vi "Dashboard Main.vi"() -> ()   [LabVIEW 2014]
uses:
  <vilib>/event_ctls.llb/eventvkey.ctl
  <vilib>/Rock Robotics/WPI/Dashboard/WPI_DashboardLogging Global.vi
  <vilib>/Rock Robotics/Network Tables/SD Write String.vi
  <vilib>/Rock Robotics/Network Tables/SD Read Number.vi
  <vilib>/Rock Robotics/Network Tables/SD Read Boolean.vi
  <vilib>/Rock Robotics/Network Tables/SD Write Boolean.vi
  <vilib>/Utility/config.llb/Write Key (String).vi
  <vilib>/Utility/config.llb/Write Key (I32).vi
  <vilib>/Utility/config.llb/NI_LVConfig.lvlib
panel:
  in  "TCP":refnum<k5>
  in  "Rec Mode":enum32{"Stop", "Record", "Playback"}(radio)
  in  "Vision":u16(ring) items=["Camera Off", "USB Camera SW", "USB Camera HW", "IP Camera"]
  out "Camera IP":string
  out "Image Message":string="Timeout in Camera Communications"
  in  "Dashboard Tab":T1(tab)
  in  "PID":bool
  in  "Camera Settings":T2={"Frame Rate"=30, "Compression"=30, "Size"=1} {"Frame Rate" scale=1.0..30.0; "Size" items=["640x480", "320x240", "160x120"]}
  out "MotorChart R":cluster{"Numeric":dbl, "Numeric":dbl}(graph)
  out "MotorChart L":T3(graph)
  out "MotorSliders R":cluster{"MotorSlide1":dbl, "MotorSlide2":dbl} {"MotorSlide2" scale=-1.0..1.0 scale format="%#_2e"; "MotorSlide1" scale=-1.0..1.0 scale format="%#_2e"}
  out "MotorSliders L":T4 {"MotorSlide4 2" scale=0.0..14.0 scale format="%#_2e"; "MotorSlide2" scale=-1.0..1.0 scale format="%#_2e"; "MotorSlide1" scale=-1.0..1.0 scale format="%#_2e"}
  out "Gyro":dbl(knob) scale=0.0..360.0
  out "JS1 Z":dbl(slide) scale=-1.0..1.0 scale format="%#_2e"
  out "JS1 Graph":cluster{"X":dbl, "Y":dbl}[](graph)
  out "JS1 Buttons":T5
  out "JS2 Z":dbl(slide) scale=-1.0..1.0 scale format="%#_2e"
  out "JS2 Graph":cluster{"X":dbl, "Y":dbl}[](graph)
  out "JS2 Buttons":T5
  out "Mode":T6(ring)=enum."Auto Disabled"
  in  "DB Camera Config":bool
  out "fps":dbl format="%#.1g"
  out "Mbps":dbl format="%#.1g"
  out "Mbps 2":bool
  out "Manual Forks?":bool
  out "PID?":bool
  in  "DB/String 9":string
  in  "DB/String 8":string
  in  "DB/String 7":string
  in  "DB/String 6":string
  in  "DB/String 5":string
  in  "DB/String 4":string
  in  "DB/String 3":string
  in  "DB/String 2":string
  in  "DB/String 1":string
  in  "DB/String 0":string
  in  "DB/Slider 0":dbl(slide) scale=0.0..5.0
  in  "DB/Slider 1":dbl(slide) scale=0.0..5.0
  in  "DB/Slider 2":dbl(slide) scale=0.0..5.0
  in  "DB/Slider 3":dbl(slide) scale=0.0..5.0
  out "DB/LED 3":bool
  out "DB/LED 2":bool
  out "DB/LED 1":bool
  out "DB/LED 0":bool
  in  "DB/Button 3":bool
  in  "DB/Button 2":bool
  in  "DB/Button 1":bool
  in  "DB/Button 0":bool caption="New Name"
  in  "AUTO Modes":T7(tab)
  in  "AUTO?":bool=TRUE
  in  "MODE":bool
  out "Totes":bool
  in  "Ring":u16(ring) items=["Left/Tote", "Left/Bin"]
  in  "Ring 2":u16(ring) items=["Center/Tote", "Center/Bin"]
  in  "Ring 3":u16(ring) items=["Right/Tote", "Right/Bin", "Right/HPS"]
  out "AUTO Zone":bool
  in  "Mode":u16(ring) items=["Drive into AUTO Zone", "Nothing"]
  in  "Test Slider":dbl(slide) scale=0.0..100.0 scale format="%#_3g"
  in  "On/Off":bool caption="Solenoid"
  in  "Test Name":u16(ring) items=["Select the test to run...", "Example Test", "-------------------------------", "List of tests is built in robot code.", "Replace with your own automated tests."]
  in  "Test Tree":string(tree)
  in  "Motor":cluster{"Value":dbl, "Enable":bool} {"Value" scale=-1.0..1.0 scale format="%#_3g"}
  out "Progress":T8 {"Test Progress" scale=0.0..100.0}
  in  "Rev/Fwd":cluster{"Forward":bool, "Reverse":bool}
  in  "Test Ring":u16(ring) items=["Monochrome", "Color"]
  in  "Listbox":i32(listbox)
  out "Tree":string(tree)
  out "Camera Image":T9(plugin-control)
  out "Boolean":bool
  # "Left"
  # "Front"
  # "Right"
  # "Battery"
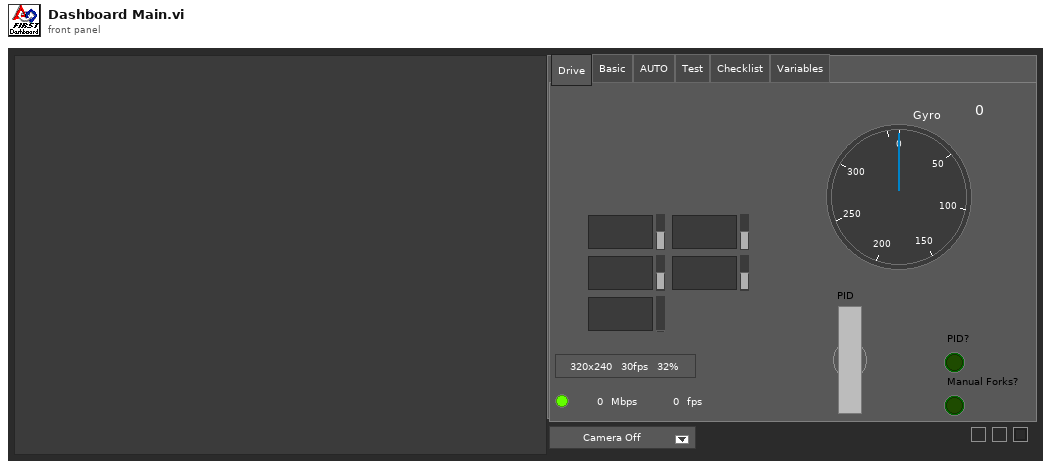
[diagram p1: front panel]
types:
  T1 = enum32{"Drive", "Basic", "AUTO", "Test", "Checklist", "Variables"}
  T2 = cluster{"Frame Rate":i32, "Compression":i32, "Size":u16}
  T3 = cluster{"Numeric":dbl, "Numeric":dbl, "Battery V":dbl}
  T4 = cluster{"MotorSlide1":dbl, "MotorSlide2":dbl, "MotorSlide4 2":dbl}
  T5 = cluster{bool, bool, bool, bool, bool, bool, bool, bool, bool, bool, bool, bool}
  T6 = enum8{"Tele-Op Disabled", "Tele-Op Enabled", "Auto Disabled", "Auto Enabled", "Test Disabled", "Test Enabled", "Disconnected", "No Code", "E-Stop"}
  T7 = enum32{"NEW USE THIS MODE", "Left", "Center", "Right", "Open Area", "Landfill"}
  T8 = cluster{"Test Progress":u8, "Test Progress Text":string}
  T9 = typedef "IMAQ Image.ctl" = refnum<image>
  T10 = enum32{"Drive", "Basic", "Custom", "Test", "Checklist", "Variables"}
  T11 = typedef "Image Type" = u32
  T12 = cluster{"Camera Image":refnum<vi>, "Dashboard Tab":refnum<vi>, "Boolean":refnum<vi>, "Vision":refnum<vi>, "Rec Mode":refnum<vi>, "Test Slider":refnum<vi>, "On/Off ":refnum<vi>, "Test Ring":refnum<vi>, "Rev/Fwd":refnum<vi>, "Test Name":refnum<vi>, "Motor":refnum<vi>, "Progress":refnum<vi>, "CheckList":refnum<vi>, "Tree":refnum<vi>, "Test Tree":refnum<vi>}
  T13 = cluster{"Error Strings":string, "Disable Counts":cluster{u16, u16}, "Rail Faults":cluster{u16, u16, u16}, "Robot IP":string, "DB Mode":u8, "Event Info":cluster{"Name":string, "Type":u8, "Number":u16, "Replay":u8}, "Camera Addr":string}
  T14 = cluster{"Storage":cluster{"Disk Free":u64, "RAM Block":u32, "RAM free":u32}, "CPU Utilization":cluster{"CPU % ISR":sgl, "CPU % Time Crit":sgl, "CPU % Timed Str":sgl, "CPU % High":sgl, "CPU % Above":sgl, "CPU % Normal":sgl, "CPU % Low":sgl}, "CAN":cluster{"% Bus Utilization":sgl, "Bus Off Cnt":u32, "TX_FIFO Full Cnt":u32, "Receive Error Cnt":u8, "Transmit Error Cnt":u8}, "HID":cluster{"HID Outputs":u32, "Rumble Low":u16, "Rumble High":u16}[]}
  T15 = cluster{"Status bits":cluster{"Test Mode":bool, "Autonomous":bool, "Enabled":bool, "Code Start":bool, "Brownout":bool, "Reserved 2":bool, "Reserved 3":bool, "E-Stop":bool}, "Code Trace":cluster{"Disabled":bool, "TeleOp":bool, "Auto":bool, "Test":bool}, "Controller Type":enum16{"unknown", "cRIO", "roboRio"}, "Code?":enum16{"unknown", "noCode", "code"}, "Battery V":dbl}
  T16 = cluster{"Control Bits":cluster{"TestMode":bool, "Autonomous":bool, "Enabled":bool, "FMS Present":bool, bool, bool, bool, "E-Stop":bool}, "Team Station ":u8, "Countdown":sgl, "Joystick Values":cluster{"Axes":dbl[], "Buttons":bool[], "POVs":i16[]}[]}
  T17 = cluster{"Axes":dbl[], "Buttons":bool[], "POVs":i16[]}[]
  T18 = cluster{"Axes":dbl[], "Buttons":bool[], "POVs":i16[]}
  T19 = cluster{"Buttons[0]":bool, "Buttons[1]":bool, "Buttons[2]":bool, "Buttons[3]":bool, "Buttons[4]":bool, "Buttons[5]":bool, "Buttons[6]":bool, "Buttons[7]":bool, "Buttons[8]":bool, "Buttons[9]":bool, "Buttons[10]":bool, "Buttons[11]":bool}
  T20 = typedef "NI_LVConfig.lvlib/Config Data RefNum.ctl" = refnum<k1>
  T21 = cluster{"Operation":enum16{"Update", "Clear"}, "Color Box":u32}[]
  T22 = typedef "eventvkey.ctl" = enum16{"ASCII", "Enter", "Return", "Shift", "Ctrl", "Alt", "Cmd", "Opt", "Caps", "NumLock", "Clear", "Break", "Up", "Down", "Left", "Right", "Insert", "Delete", "Home", "End", "PageUp", "PageDown", "Escape", "Help", "Pause", "ScrollLock", "F1", "F2", "F3", "F4", "F5", "F6", "F7", "F8", "F9", "F10", "F11", "F12", "F13", "F14", "F15", "F16", "F17", "F18", "F19", "F20", "F21", "F22", "F23", "F24", "Play", "VolumeUp", "VolumeDown", "Mute", "Two Byte Char"}
  T23 = cluster{"Image Size":bool, "Image Type":bool, "Pixel Value":bool, "ROI Information":bool, "Zoom Factor":bool}
  T24 = enum8{"Enabled", "Disabled", "Disabled and Grayed Out"}
  T25 = cluster{"Operation":enum16{"Update", "Clear"}, "Color Box":u32}
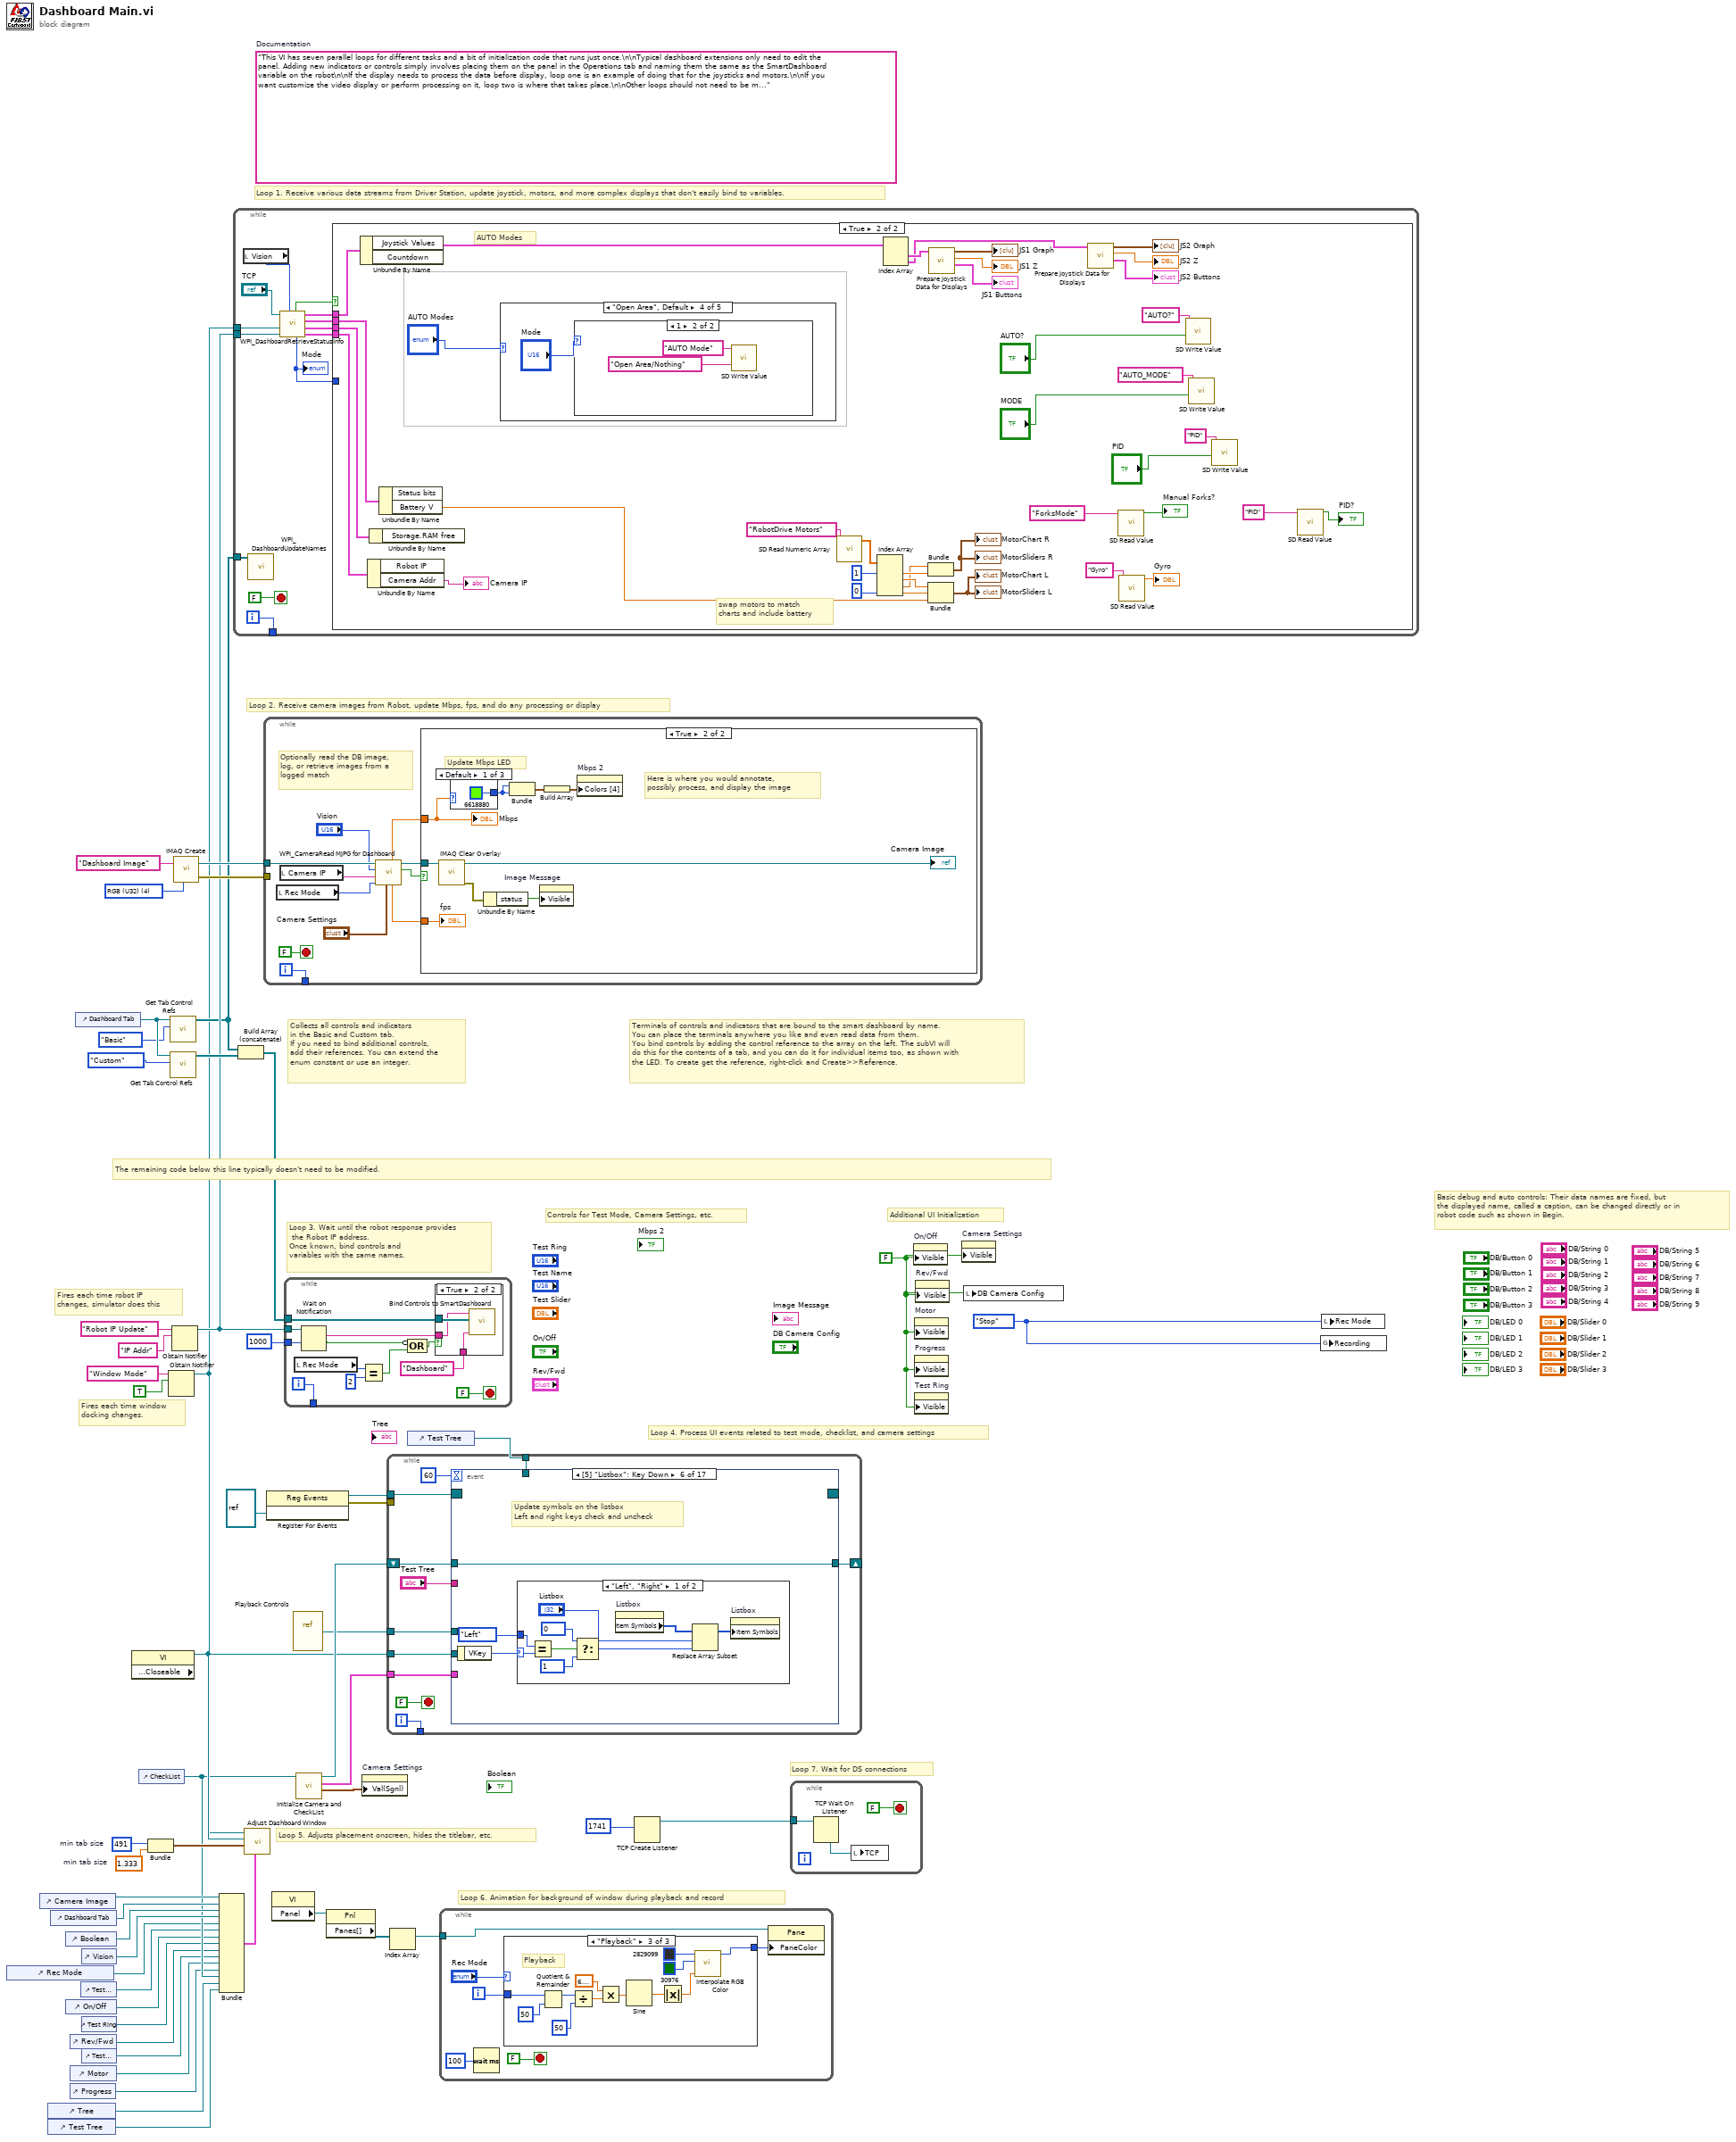
[diagram p0: block diagram]
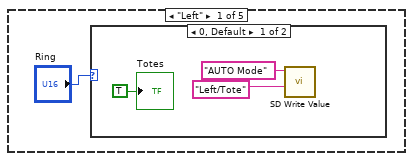
[diagram p3: hidden frame]
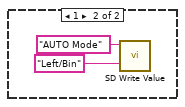
[diagram p4: hidden frame]
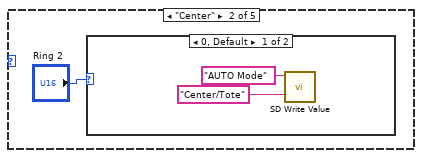
[diagram p5: hidden frame]
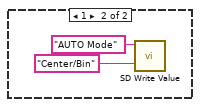
[diagram p6: hidden frame]
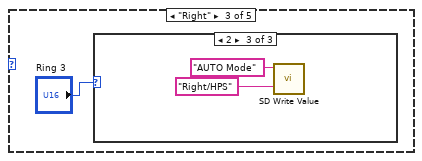
[diagram p7: hidden frame]
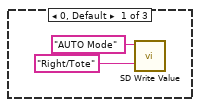
[diagram p8: hidden frame]
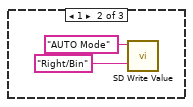
[diagram p9: hidden frame]
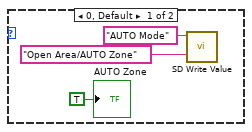
[diagram p10: hidden frame]
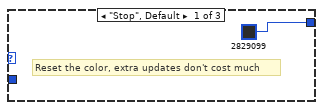
[diagram p12: hidden frame]
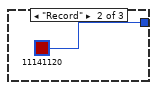
[diagram p13: hidden frame]
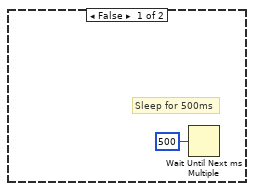
[diagram p15: hidden frame]
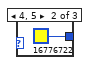
[diagram p16: hidden frame]
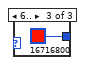
[diagram p17: hidden frame]
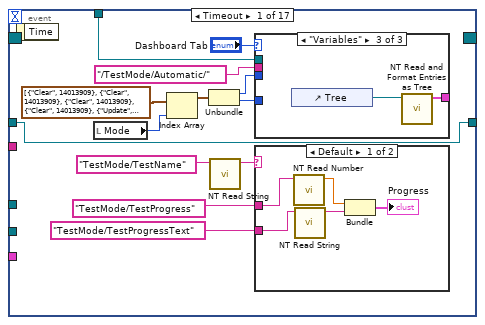
[diagram p18: hidden frame]
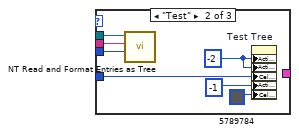
[diagram p20: hidden frame]
diagram:
  w24 = 491  # min tab size
  w23 = 1.333  # min tab size
  w32 = enum32{"Stop", "Record", "Playback"}."Stop" ("Rec Mode")
  w6 = FALSE ("Visible")
  (unwired) "This VI has seven parallel loops for different tasks and a bit of initialization code that runs just once.\n\nTypical dashboard extensions only need to edit the panel. Adding new indicators or controls simply involves placing them on the panel in the Operations tab and naming them the same as the SmartDashboard variable on the robot\n\nIf the display needs to process the data before display, loop one is an example of doing that for the joysticks and motors.\n\nIf you want customize the video display or perform processing on it, loop two is where that takes place.\n\nOther loops should not need to be modified. They are pretty standard, and document the task they perform."  # Documentation
  w52 = T11 4 items=["Grayscale (U8)", "Grayscale (I16)", "Grayscale (SGL)", "Complex (CSG)", "RGB (U32)", "HSL (U32)", "RGB (U64)"] ("Image Type")
  # "Loop 7. Wait for DS connections"
  # "Basic debug and auto controls: Their data names are fixed, but\nthe displayed name, called a caption, can be changed directly or in\nrobot code such as shown in Begin."
  # "Controls for Test Mode, Camera Settings, etc."
  # "Additional UI Initialization"
  # "Loop 6. Animation for background of window during playback and record"
  # "Fires each time robot IP\nchanges, simulator does this"
  # "Fires each time window\ndocking changes."
  # "Collects all controls and indicators\nin the Basic and Custom tab.\nIf you need to bind additional controls,\nadd their references. You can extend the\nenum constant or use an integer."
  # "The remaining code below this line typically doesn't need to be modified."
  # "Loop 4. Process UI events related to test mode, checklist, and camera settings"
  # "Terminals of controls and indicators that are bound to the smart dashboard by name.\nYou can place the terminals anywhere you like and even read data from them.\nYou bind controls by adding the control reference to the array on the left. The subVI will\ndo this for the contents of a tab, and you can do it for individual items too, as shown with\nthe LED. To create get the reference, right-click and Create>>Reference."
  # "Loop 3. Wait until the robot response provides\n the Robot IP address.\nOnce known, bind controls and\nvariables with the same names."
  # "Loop 5. Adjusts placement onscreen, hides the titlebar, etc."
  # "Loop 1. Receive various data streams from Driver Station, update joystick, motors, and more complex displays that don't easily bind to variables."
  # "Loop 2. Receive camera images from Robot, update Mbps, fps, and do any processing or display"
  n1 = control-ref of="Rec Mode"() -> (w12:refnum<vi>)
  n2 = control-ref of="Camera Image"() -> (w27:refnum<vi>)
  n3 = control-ref of="Tree"() -> (w16:refnum<vi>)
  n4 = control-ref of="Test Tree"() -> (w15:refnum<vi>)
  n5 = control-ref of="Dashboard Tab"() -> (w26:refnum<vi>)
  n6 = control-ref of="Boolean"() -> (w21:refnum<vi>)
  n7 = control-ref of="On/Off"() -> (w10:refnum<vi>)
  n8 = control-ref of="Progress"() -> (w7:refnum<vi>)
  n9 = control-ref of="Rev/Fwd"() -> (w8:refnum<vi>)
  n10 = control-ref of="Motor"() -> (w13:refnum<vi>)
  n11 = control-ref of="Dashboard Tab"() -> (w30:refnum<vi>)
  n12 = control-ref of="Test Slider"() -> (w11:refnum<vi>)
  n13 = control-ref of="Vision"() -> (w25:refnum<vi>)
  n14 = control-ref of="Test Ring"() -> (w9:refnum<vi>)
  n15 = control-ref of="Test Name"() -> (w14:refnum<vi>)
  n16 = property class="VI" props=["Front Panel.Closeable"]() -> (reference out=w31:refnum<vi>)  [unwired: 2 in, 2 out]
  n17 = control-ref of="CheckList"() -> (w17:refnum<vi>)
  n18 = Bundle("min tab size"=w24, "min tab size"=w23) -> (w22:cluster{"min tab size":i32, "min tab size":dbl})  [unwired: 1 in]
  n19 = Obtain Notifier(name (unnamed)="Window Mode", notification data type=TRUE) -> (notifier out=w3:refnum<notifier>)  [unwired: 2 in, 2 out]
  n20 = call <vilib>:"Get Tab Control Refs.vi"("Page Index"=T10."Basic" ("Dashboard Tab"), "TabControl in"=w30) -> ("ControlsOnPage"=w4:refnum<vi>[])  [unwired: 9 in]
  n21 = call <vilib>:"Get Tab Control Refs.vi"("Page Index"=T10."Custom" ("Dashboard Tab"), "TabControl in"=w30) -> ("ControlsOnPage"=w29:refnum<vi>[])  [unwired: 9 in]
  n22 = Obtain Notifier(name (unnamed)="Robot IP Update", notification data type="IP Addr" ("name (unnamed)")) -> (notifier out=w5:refnum<notifier>)  [unwired: 2 in, 2 out]
  n23 = call "IMAQ Create"("Image Name"="Dashboard Image", "Image Type"=w52) -> ("New Image"=w50:T9, "error out"=w49:errorcluster)  [unwired: 2 in, 1 out]
  n24 = Bundle("Camera Image"=w27, "Dashboard Tab"=w26, "Boolean"=w21, "Vision"=w25, "Rec Mode"=w12, "Test Slider"=w11, "On/Off"=w10, "Test Ring"=w9, "Rev/Fwd"=w8, "Test Name"=w14, "Motor"=w13, "Progress"=w7, "CheckList"=w17, "Tree"=w16, "Test Tree"=w15) -> (w18:T12)  [unwired: 1 in]
  n25 = while {
    tunnel: [w64] -> _
    tunnel: w5 -> [w58]
    tunnel: w4 -> [w57]
    tunnel: w3 -> [w53]
    i -> [w64]
    stop <- FALSE stop-if-true
    n26 = local read "Vision"() -> (w55:u16)
    n27 = call <vilib>:"WPI_DashboardUpdateNames.vi"("Controls on Tab"=w57) -> ()  [unwired: 11 in]
    n28 = call <vilib>:"WPI_DashboardRetrieveStatusInfo.vi"("Vision"=w55, "Binding Refnum"=w58, "Window Mode Notifier"=w53, "TCP Cnx"="TCP") -> ("Power and Errors"=w59:T13, "Robot Metrics"=w62:T14, "Status Info"=w63:T15, "Control Info"=w60:T16, "Robot Mode"=w56:T6, "Process?"=w61:bool)  [unwired: 2 in]
    "Mode" <- w56
    n29 = case shown="True" w61 {
      tunnel: w63 -> [_ w103]
      tunnel: w62 -> [_ w102]
      tunnel: w60 -> [_ w101]
      tunnel: w59 -> [_ w100]
      tunnel: w56 -> [_ _]
      frame False {
      }
      frame True {
        # "AUTO Modes"
        # "swap motors to match\ncharts and include battery"
        n30 = Unbundle By Name(w101) -> ("Joystick Values"=w88:T17)  [unwired: 1 out]
        n31 = Unbundle By Name(w100) -> ("Camera Addr"=→"Camera IP":string)  [unwired: 1 out]
        n32 = Unbundle By Name(w102) -> ()  [unwired: 1 out]
        n33 = Unbundle By Name(w103) -> ("Battery V"=w89:dbl)  [unwired: 1 out]
        n34 = case shown="\"Open Area\", Default" "AUTO Modes" {
          frame "Left" {
            n35 = case shown="0, Default" "Ring" {
              frame 0, Default {
                n36 = call-poly <vilib>:"SD Write Value.vi"("String"="Left/Tote", "Name"="AUTO Mode") -> ()  [unwired: 8 in, 2 out]
                "Totes" <- TRUE ("Totes")
              }
              frame 1 {
                n37 = call-poly <vilib>:"SD Write Value.vi"("String"="Left/Bin", "Name"="AUTO Mode") -> ()  [unwired: 8 in, 2 out]
              }
            }
          }
          frame "Center" {
            n38 = case shown="0, Default" "Ring 2" {
              frame 0, Default {
                n39 = call-poly <vilib>:"SD Write Value.vi"("String"="Center/Tote", "Name"="AUTO Mode") -> ()  [unwired: 8 in, 2 out]
              }
              frame 1 {
                n40 = call-poly <vilib>:"SD Write Value.vi"("String"="Center/Bin", "Name"="AUTO Mode") -> ()  [unwired: 8 in, 2 out]
              }
            }
          }
          frame "Right" {
            n41 = case shown="2" "Ring 3" {
              frame 0, Default {
                n42 = call-poly <vilib>:"SD Write Value.vi"("String"="Right/Tote", "Name"="AUTO Mode") -> ()  [unwired: 8 in, 2 out]
              }
              frame 1 {
                n43 = call-poly <vilib>:"SD Write Value.vi"("String"="Right/Bin", "Name"="AUTO Mode") -> ()  [unwired: 8 in, 2 out]
              }
              frame 2 {
                n44 = call-poly <vilib>:"SD Write Value.vi"("String"="Right/HPS", "Name"="AUTO Mode") -> ()  [unwired: 8 in, 2 out]
              }
            }
          }
          frame "Open Area", Default {
            n45 = case shown="1" "Mode" {
              frame 0, Default {
                n46 = call-poly <vilib>:"SD Write Value.vi"("String"="Open Area/AUTO Zone", "Name"="AUTO Mode") -> ()  [unwired: 8 in, 2 out]
                "AUTO Zone" <- TRUE ("AUTO Zone")
              }
              frame 1 {
                n47 = call-poly <vilib>:"SD Write Value.vi"("String"="Open Area/Nothing", "Name"="AUTO Mode") -> ()  [unwired: 8 in, 2 out]
              }
            }
          }
          frame "Landfill" {
          }
        }
        n48 = call <vilib>:"SD Read Numeric Array.vi"("Name"="RobotDrive Motors") -> ("Numeric Array"=w91:dbl[])  [unwired: 8 in, 2 out]
        n49 = Index Array(array=w91, index #1=1, index #4=0) -> (element #1=w95:dbl, element #2=w96:dbl, element #3=w94:dbl, element #4=w99:dbl)  [unwired: 2 in]
        n50 = Index Array(array=w88) -> (element #1=w87:T18, element #2=w82:T18)  [unwired: 2 in]
        n51 = Bundle("Numeric"=w94, "Numeric"=w95) -> (→"MotorChart R" →"MotorSliders R":cluster{"Numeric":dbl, "Numeric":dbl})  [unwired: 1 in]
        n52 = Bundle("Numeric"=w96, "Numeric"=w99, "Battery V"=w89) -> (→"MotorChart L" →"MotorSliders L":T3)  [unwired: 1 in]
        n53 = call "Prepare Joystick Data for Displays.vi"("Joystick Values"=w87) -> ("Buttons"=→"JS1 Buttons":T19, "Z Axis"=→"JS1 Z":dbl, "Cartesian Data"=→"JS1 Graph":cluster{"X axis":dbl, "X axis":dbl}[])  [unwired: 8 in]
        n54 = call "Prepare Joystick Data for Displays.vi"("Joystick Values"=w82) -> ("Buttons"=→"JS2 Buttons":T19, "Z Axis"=→"JS2 Z":dbl, "Cartesian Data"=→"JS2 Graph":cluster{"X axis":dbl, "X axis":dbl}[])  [unwired: 8 in]
        n55 = call-poly <vilib>:"SD Read Value.vi"("Name"="ForksMode") -> ("Boolean"=→"Manual Forks?":bool)  [unwired: 8 in, 2 out]
        n56 = call-poly <vilib>:"SD Read Value.vi"("Name"="Gyro") -> ("Numeric"=→"Gyro":dbl)  [unwired: 8 in, 2 out]
        n57 = call-poly <vilib>:"SD Write Value.vi"("Boolean"="AUTO?", "Name"="AUTO?") -> ()  [unwired: 8 in, 2 out]
        n58 = call-poly <vilib>:"SD Write Value.vi"("Boolean"="MODE", "Name"="AUTO_MODE") -> ()  [unwired: 8 in, 2 out]
        n59 = call-poly <vilib>:"SD Write Value.vi"("Boolean"="PID", "Name"="PID") -> ()  [unwired: 8 in, 2 out]
        n60 = call-poly <vilib>:"SD Read Value.vi"("Name"="PID") -> ("Boolean"=→"PID?":bool)  [unwired: 8 in, 2 out]
      }
    }
  }
  n61 = Build Array (concatenate)(w4, w29) -> (w28:refnum<vi>[])
  n62 = call "Adjust Dashboard Window.vi"("Sizing Refnums"=w18, "Size Constraints"=w22, "VI"=w31, "Notifier in"=w3) -> ()  [unwired: 8 in]
  n63 = while {
    tunnel: w50 -> [w136]
    tunnel: w49 -> [_]
    tunnel: [w137] -> _
    i -> [w137]
    stop <- FALSE stop-if-true
    # "Optionally read the DB image,\nlog, or retrieve images from a\nlogged match"
    n64 = local read "Rec Mode"() -> (w130:enum32{"Stop", "Record", "Playback"})
    n65 = local read "Camera IP"() -> (w128:string)
    n66 = call <vilib>:"WPI_CameraRead MJPG for Dashboard.vi"("Camera Settings"="Camera Settings", "Rec Mode"=w130, "Camera IP"=w128, "Camera Mode"="Vision", "Refnum in"=w136) -> ("Active"=w134:bool, "Refnum out"=w135:T9, "FPS"=w133:dbl, "Bandwidth (Mbps)"=w132:dbl)  [unwired: 3 in]
    n67 = case shown="True" w134 {
      tunnel: w135 -> [_ w143]
      tunnel: w132 -> [_ w142]
      tunnel: w133 -> [_ w140]
      frame False {
        # "Sleep for 500ms"
        n68 = Wait Until Next ms Multiple(millisecond multiple=u32 500) -> ()  [unwired: 1 out]
      }
      frame True {
        # "Here is where you would annotate,\npossibly process, and display the image"
        # "Update Mbps LED"
        n69 = call "IMAQ Clear Overlay"("Image"=w143) -> ("error out"=w147:errorcluster, "Image Out"=→"Camera Image":T9)  [unwired: 2 in, 7 out]
        n70 = case shown="Default" w142 {
          tunnel: [u32 6618880 ("Color Box") u32 16776722 ("Color Box") u32 16716800 ("Color Box")] -> w144
          frame Default {
          }
          frame 4, 5 {
          }
          frame 6.. {
          }
        }
        n71 = Unbundle By Name(w147) -> ("status"=w148:bool)
        n72 = Bundle("Color Box"=w144, "Color Box"=w144) -> (w146:cluster{"Color Box":u32, "Color Box":u32})  [unwired: 1 out]
        n73 = property on="Image Message" class="Str"("Visible"=w148) -> ()  [unwired: 2 in, 2 out]
        n74 = Build Array(w146) -> (w145:cluster{"Color Box":u32, "Color Box":u32}[])
        n75 = property on="Mbps 2" class="Bool (strict)"("Colors [4]"=w145) -> ()  [unwired: 2 in, 2 out]
        "Mbps" <- w142
        "fps" <- w140
      }
    }
  }
  n76 = register-events(refnum<vi> refnum) -> (reference out=w36:refnum<event-registration>, error out=w35:errorcluster)  [unwired: 2 in]
  n77 = property class="VI"() -> ("Panel"=w39:refnum<vi>)  [unwired: 2 in, 2 out]
  n78 = while {
    tunnel: w28 -> [w163]
    tunnel: w5 -> [w161]
    tunnel: [w159] -> _
    tunnel: u32 1000 ("milliseconds to wait") -> [w158]
    i -> [w159]
    stop <- FALSE stop-if-true
    n79 = local read "Rec Mode"() -> (w154:enum32{"Stop", "Record", "Playback"})
    n80 = Wait on Notification(notifier=w161, timeout in ms (-1)=w158) -> (notification=w160:string, timed out?=w156:bool)  [unwired: 2 in, 2 out]
    n81 = Equal?(x=w154, y=u16 2 ("Rec Mode")) -> (x = y?=w155:bool)
    n82 = Compound Arithmetic op=OR(invert w156, w155) -> (w157:bool)
    n83 = case shown="True" w157 {
      tunnel: w163 -> [_ w166]
      tunnel: w160 -> [_ w165]
      tunnel: "Dashboard" -> [_ w164]
      frame False {
      }
      frame True {
        n84 = call <vilib>:"Bind Controls to SmartDashboard.vi"("Client Name"=w164, "Bound Control Refs"=w166, "Server IP Address"=w165) -> ()  [unwired: 9 in]
      }
    }
  }
  n85 = vi-ref "Playback Controls.vi"() -> (w37:refnum<vi>)
  n86 = call "Initialize Camera and CheckList.vi"("ListBox in"=w17) -> ("Cluster"=w43:cluster{"value":i32, "value":i32, "index":i32}, "Array"=w44:cluster{string[]}[], "File Refnum"=w42:T20)  [unwired: 8 in]
  n87 = property class="Pnl"(reference=w39) -> ("Panes[]"=w40:refnum<vi>[])  [unwired: 1 in, 2 out]
  n88 = property on="Camera Settings" class="Clust (strict)"("Val(Sgnl)"=w43) -> ()  [unwired: 2 in, 2 out]
  n89 = Index Array(array=w40) -> (element=w38:refnum<vi>)  [unwired: 1 in]
  n90 = control-ref of="Test Tree"() -> (w41:refnum<vi>)
  n91 = while {
    tunnel: w44 -> [w174]
    shift-right: [w173] -> _
    shift-left: w42 -> [w172]
    tunnel: [w171] -> _
    tunnel: w41 -> [w170]
    tunnel: w37 -> [w169]
    tunnel: w36 -> [w168]
    tunnel: w35 -> [_]
    tunnel: w31 -> [w167]
    i -> [w171]
    stop <- FALSE stop-if-true
    n92 = event shown="[5] \"Listbox\": Key Down" {
      selector: w168 -> [_ _ _ _ _ _ _ _ _ _ _ _ _ _ _ _ _]
      dyn-events: [_ _ _ _ _ _ _ _ _ _ _ _ _ w412 _ _ _] -> _
      timeout: u32 60 ("milliseconds to wait") -> [_ _ _ _ _ _ _ _ _ _ _ _ _ _ _ _ _]
      tunnel: w170 -> [w186 _ _ _ _ _ _ _ _ _ _ _ _ _ _ _ _]
      tunnel: "Test Tree" -> [_ _ _ _ _ _ _ _ w381 w389 w391 w395 w403 _ _ _ _]
      tunnel: w174 -> [_ w208 _ _ _ _ w345 w375 _ _ _ _ _ _ _ _ _]
      tunnel: [w182 w207 w306 w311 w319 w331 w344 w368 w380 w387 w390 w394 w402 w414 w428 w429 w439] -> w173
      tunnel: w172 -> [w182 w207 w306 w311 w319 w331 w343 w368 w380 w387 w390 w394 w402 w414 w428 w429 w439]
      tunnel: w169 -> [_ _ _ _ _ _ _ _ _ _ _ _ _ w415 _ w432 _]
      tunnel: w167 -> [_ _ _ _ _ _ _ _ _ _ _ _ _ w410 _ _ _]
      event Timeout {
        n93 = event-data() -> ()  [unwired: 1 in, 1 out]
        n94 = local read "Mode"() -> (w185:T6)
        n95 = Index Array(array=T21 [{"Operation"=enum."Clear", "Color Box"=14013909}, {"Operation"=enum."Clear", "Color Box"=14013909}, {"Operation"=enum."Clear", "Color Box"=14013909}, {"Operation"=enum."Clear", "Color Box"=14013909}, {"Operation"=enum."Update", "Color Box"=14013909}, {"Operation"=enum."Update", "Color Box"=16777215}, {"Operation"=enum."Clear", "Color Box"=14013909}, {"Operation"=enum."Clear", "Color Box"=14013909}, {"Operation"=enum."Clear", "Color Box"=14013909}], index=w185) -> (element=w180:T25)
        n96 = Unbundle(w180) -> ("Operation"=w179:enum16{"Update", "Clear"}, "Color Box"=w178:u32)
        n97 = call <vilib>:"NT Read String.vi"("Name"="TestMode/TestName") -> ("String"=w189:string)  [unwired: 9 in, 1 out]
        n98 = case shown="\"Variables\"" "Dashboard Tab" {
          tunnel: w186 -> [_ w197 _]
          tunnel: "/TestMode/Automatic/" ("Name Pattern") -> [_ w196 _]
          tunnel: w179 -> [_ w195 _]
          tunnel: [_ _ w199] -> _
          tunnel: w178 -> [_ w191 _]
          frame "AUTO", Default {
          }
          frame "Test" {
            w194 = -2 ("Active Item:Row Number")
            n99 = call <vilib>:"NT Read and Format Entries as Tree.vi"("Operation"=w195, "Name Pattern"=w196, "Tree Refnum"=w197) -> ()  [unwired: 7 in, 2 out]
            n100 = property on="Test Tree" class="Tree (strict)"("Active Item Row Number"=w194, "ActiveColNum"=w194, "CellBG"=w191, "Active Item Row Number"=-1 ("Active Item:Row Number"), "CellBG"=u32 5789784 ("Color Box")) -> ()  [unwired: 2 in, 2 out]
          }
          frame "Variables" {
            n101 = control-ref of="Tree"() -> (w198:refnum<vi>)
            n102 = call <vilib>:"NT Read and Format Entries as Tree.vi"("Tree Refnum"=w198) -> ("Formatted Strings"=w199:cluster{"Name":string, "Value":string}[])  [unwired: 9 in, 1 out]
          }
        }
        n103 = case shown="Default" w189 {
          tunnel: "TestMode/TestProgress" ("Name") -> [w201 _]
          tunnel: "TestMode/TestProgressText" ("Name") -> [w200 _]
          frame Default {
            n104 = call <vilib>:"NT Read Number.vi"("Name"=w201) -> ("Numeric"=w202:dbl)  [unwired: 9 in, 1 out]
            n105 = call <vilib>:"NT Read String.vi"("Name"=w200) -> ("String"=w203:string)  [unwired: 9 in, 1 out]
            n106 = Bundle("Numeric"=w202, "String"=w203) -> (→"Progress":cluster{"Numeric":dbl, "String":string})  [unwired: 1 in]
          }
          frame "" {
            n107 = property on="Progress" class="Clust (strict)"("Visible"=FALSE) -> ()  [unwired: 2 in, 2 out]
            n108 = local write "Test Name"(u16 0) -> ()
          }
        }
      }
      event "Test Tree": Value Change {
        # "Show appropriate\ncontrols"
        n109 = event-data() -> ("CtlRef"=w211:refnum<vi>, "NewVal"=w209:string)  [unwired: 1 in]
        n110 = call <vilib>:"WPI_UtilitiesGetTreeIOName.vi"("NewVal"=w209, "TreeControl in"=w211) -> ("I/O Name"=w212:string)  [unwired: 9 in]
        n111 = case shown="\"Camera\"" w212 {
          selector: w212 -> [_ w219 _ w237 w246 _]
          tunnel: w209 -> [_ _ w234 w236 _ w253]
          tunnel: w208 -> [_ _ _ _ _ w252]
          frame Default {
            w214 = FALSE ("Visible")
            w213 = FALSE ("Visible")
            n112 = property on="Motor" class="Clust (strict)"("Visible"=w213) -> ()  [unwired: 2 in, 2 out]
            n113 = property on="Test Ring" class="Ring (strict)"("Visible"=w213) -> ()  [unwired: 2 in, 2 out]
            n114 = property on="Rev/Fwd" class="Clust (strict)"("Visible"=w214) -> ()  [unwired: 2 in, 2 out]
            n115 = property on="On/Off" class="Bool (strict)"("Visible"=w214) -> ()  [unwired: 2 in, 2 out]
            n116 = property on="Test Slider" class="Slide (strict)"("Visible"=w214) -> ()  [unwired: 2 in, 2 out]
          }
          frame "Motor", "PWM" {
            w220 = FALSE ("Visible")
            n117 = case shown="\"Motor\", Default" w219 {
              tunnel: [1.0 ("Value") -1.0 ("Value")] -> w218
              tunnel: [255.0 ("Value") 1.0 ("Value")] -> w217
              tunnel: [128.0 ("Value") 0.0 ("Value")] -> w216
              tunnel: [64.0 ("Value") 0.5 ("Value")] -> w215
              frame "PWM" {
              }
              frame "Motor", Default {
              }
            }
            n118 = property on="Motor" class="Clust (strict)"("Visible"=TRUE) -> ()  [unwired: 2 in, 2 out]
            n119 = property on="Value" class="Slide (strict)"("Value"=w216, "Scale.Minimum"=w218, "Scale.Maximum"=w217, "Scale.Increment"=w215) -> ()  [unwired: 2 in, 2 out]
            n120 = property on="On/Off" class="Bool (strict)"("Visible"=w220) -> ()  [unwired: 2 in, 2 out]
            n121 = property on="Test Slider" class="Slide (strict)"("Visible"=w220) -> ()  [unwired: 2 in, 2 out]
            n122 = property on="Test Ring" class="Ring (strict)"("Visible"=w220) -> ()  [unwired: 2 in, 2 out]
            n123 = property on="Rev/Fwd" class="Clust (strict)"("Visible"=w220) -> ()  [unwired: 2 in, 2 out]
          }
          frame "Servo" {
            w232 = FALSE ("Visible")
            n124 = call <vilib>:"NT Read Number.vi"("Name"=w234) -> ("Numeric"=w233:dbl)  [unwired: 9 in, 1 out]
            n125 = property on="Test Slider" class="Slide (strict)"("Visible"=TRUE, "Scale.Maximum"=170.0 ("Scale.Range:Maximum")) -> ()  [unwired: 2 in, 2 out]
            n126 = local write "Test Slider"(w233) -> ()
            n127 = property on="Motor" class="Clust (strict)"("Visible"=w232) -> ()  [unwired: 2 in, 2 out]
            n128 = property on="Rev/Fwd" class="Clust (strict)"("Visible"=w232) -> ()  [unwired: 2 in, 2 out]
            n129 = property on="On/Off" class="Bool (strict)"("Visible"=w232) -> ()  [unwired: 2 in, 2 out]
            n130 = property on="Test Ring" class="Ring (strict)"("Visible"=w232) -> ()  [unwired: 2 in, 2 out]
          }
          frame "Relay", "Solenoid" {
            w235 = FALSE ("Visible")
            n131 = property on="Motor" class="Clust (strict)"("Visible"=w235) -> ()  [unwired: 2 in, 2 out]
            n132 = property on="Test Slider" class="Slide (strict)"("Visible"=w235) -> ()  [unwired: 2 in, 2 out]
            n133 = Search and Replace String(input string=w236, search string="/Value  **", replace string="/Direction") -> (result string=w242:string)  [unwired: 5 in, 3 out]
            n134 = property on="Test Ring" class="Ring (strict)"("Visible"=w235) -> ()  [unwired: 2 in, 2 out]
            n135 = call <vilib>:"NT Read String.vi"("Name"=w242) -> ("String"=w240:string)  [unwired: 9 in, 1 out]
            n136 = Equal?(x="Both directions", y=w240) -> (x = y?=w238:bool)
            n137 = Not(x=w238) -> (.not. x?=w239:bool)
            n138 = property on="Rev/Fwd" class="Clust (strict)"("Visible"=w238) -> ()  [unwired: 2 in, 2 out]
            n139 = property on="On/Off" class="Bool (strict)"("Visible"=w239, "Caption.Text"=w237) -> ()  [unwired: 2 in, 2 out]
          }
          frame "Compressor", "Digital Out" {
            w245 = FALSE ("Visible")
            # "Get direction and finish"
            n140 = property on="Motor" class="Clust (strict)"("Visible"=w245) -> ()  [unwired: 2 in, 2 out]
            n141 = property on="Test Slider" class="Slide (strict)"("Visible"=w245) -> ()  [unwired: 2 in, 2 out]
            n142 = property on="Test Ring" class="Ring (strict)"("Visible"=w245) -> ()  [unwired: 2 in, 2 out]
            n143 = property on="On/Off" class="Bool (strict)"("Visible"=TRUE, "Caption.Text"=w246) -> ()  [unwired: 2 in, 2 out]
            n144 = property on="Rev/Fwd" class="Clust (strict)"("Visible"=FALSE) -> ()  [unwired: 2 in, 2 out]
          }
          frame "Camera" {
            n145 = call <vilib>:"Get Last Path Segment.vi"("String in"=w253) -> ("String out"=w254:string)  [unwired: 10 in]
            n146 = property on="On/Off" class="Bool (strict)"("Visible"=FALSE) -> ()  [unwired: 2 in, 2 out]
            n147 = property on="Motor" class="Clust (strict)"("Visible"=FALSE) -> ()  [unwired: 2 in, 2 out]
            n148 = property on="Rev/Fwd" class="Clust (strict)"("Visible"=FALSE) -> ()  [unwired: 2 in, 2 out]
            n149 = case shown="\"White Balance  **\"" w254 {
              tunnel: w253 -> [w260 w269 w278 w287 w296 _ w302]
              tunnel: w252 -> [w258 w266 w275 w284 w293 _ _]
              frame "Size  **" {
                n150 = Index Array(array=w258) -> (element=w257:cluster{string[]})  [unwired: 1 in]
                n151 = call <vilib>:"NT Read String.vi"("Name"=w260) -> ("String"=w259:string)  [unwired: 9 in, 1 out]
                n152 = Unbundle(w257) -> (w255:string[])
                n153 = Match First String(2:w255, 3:w259) -> (0:w256:i32)  [unwired: 1 out]
                n154 = property on="Test Ring" class="Ring (strict)"("Value"=w256, "Strings []"=w255) -> ()  [unwired: 2 in, 2 out]
                n155 = property on="Test Ring" class="Ring (strict)"("Visible"=TRUE) -> ()  [unwired: 2 in, 2 out]
                n156 = property on="Test Slider" class="Slide (strict)"("Visible"=FALSE) -> ()  [unwired: 2 in, 2 out]
              }
              frame "White Balance  **" {
                n157 = Index Array(array=w266, index=1) -> (element=w267:cluster{string[]})
                n158 = call <vilib>:"NT Read String.vi"("Name"=w269) -> ("String"=w268:string)  [unwired: 9 in, 1 out]
                n159 = Unbundle(w267) -> (w264:string[])
                n160 = Match First String(2:w264, 3:w268) -> (0:w263:i32)  [unwired: 1 out]
                n161 = property on="Test Ring" class="Ring (strict)"("Value"=w263, "Strings []"=w264) -> ()  [unwired: 2 in, 2 out]
                n162 = property on="Test Ring" class="Ring (strict)"("Visible"=TRUE) -> ()  [unwired: 2 in, 2 out]
                n163 = property on="Test Slider" class="Slide (strict)"("Visible"=FALSE) -> ()  [unwired: 2 in, 2 out]
              }
              frame "Exposure  **" {
                n164 = Index Array(array=w275, index=2) -> (element=w276:cluster{string[]})
                n165 = call <vilib>:"NT Read String.vi"("Name"=w278) -> ("String"=w277:string)  [unwired: 9 in, 1 out]
                n166 = Unbundle(w276) -> (w272:string[])
                n167 = Match First String(2:w272, 3:w277) -> (0:w273:i32)  [unwired: 1 out]
                n168 = property on="Test Ring" class="Ring (strict)"("Value"=w273, "Strings []"=w272) -> ()  [unwired: 2 in, 2 out]
                n169 = property on="Test Ring" class="Ring (strict)"("Visible"=TRUE) -> ()  [unwired: 2 in, 2 out]
                n170 = property on="Test Slider" class="Slide (strict)"("Visible"=FALSE) -> ()  [unwired: 2 in, 2 out]
              }
              frame "Exposure Priority  **" {
                n171 = Index Array(array=w284, index=3) -> (element=w285:cluster{string[]})
                n172 = call <vilib>:"NT Read String.vi"("Name"=w287) -> ("String"=w286:string)  [unwired: 9 in, 1 out]
                n173 = Unbundle(w285) -> (w281:string[])
                n174 = Match First String(2:w281, 3:w286) -> (0:w282:i32)  [unwired: 1 out]
                n175 = property on="Test Ring" class="Ring (strict)"("Value"=w282, "Strings []"=w281) -> ()  [unwired: 2 in, 2 out]
                n176 = property on="Test Ring" class="Ring (strict)"("Visible"=TRUE) -> ()  [unwired: 2 in, 2 out]
                n177 = property on="Test Slider" class="Slide (strict)"("Visible"=FALSE) -> ()  [unwired: 2 in, 2 out]
              }
              frame "Color Enable  **" {
                n178 = Index Array(array=w293, index=4) -> (element=w294:cluster{string[]})
                n179 = call <vilib>:"NT Read String.vi"("Name"=w296) -> ("String"=w295:string)  [unwired: 9 in, 1 out]
                n180 = Unbundle(w294) -> (w290:string[])
                n181 = Match First String(2:w290, 3:w295) -> (0:w291:i32)  [unwired: 1 out]
                n182 = property on="Test Ring" class="Ring (strict)"("Value"=w291, "Strings []"=w290) -> ()  [unwired: 2 in, 2 out]
                n183 = property on="Test Ring" class="Ring (strict)"("Visible"=TRUE) -> ()  [unwired: 2 in, 2 out]
                n184 = property on="Test Slider" class="Slide (strict)"("Visible"=FALSE) -> ()  [unwired: 2 in, 2 out]
              }
              frame Default {
                n185 = property on="Test Ring" class="Ring (strict)"("Visible"=FALSE) -> ()  [unwired: 2 in, 2 out]
                n186 = property on="Test Slider" class="Slide (strict)"("Visible"=FALSE) -> ()  [unwired: 2 in, 2 out]
              }
              frame "Brightness  **", "Color Level  **", "Compression  **", "FPS  **", "Sharpness  **" {
                n187 = call <vilib>:"NT Read Number.vi"("Name"=w302) -> ("Numeric"=w301:dbl)  [unwired: 9 in, 1 out]
                n188 = local write "Test Slider"(w301) -> ()
                n189 = property on="Test Slider" class="Slide (strict)"("Visible"=TRUE, "Scale.Maximum"=100.0 ("Scale.Range:Maximum")) -> ()  [unwired: 2 in, 2 out]
                n190 = property on="Test Ring" class="Ring (strict)"("Visible"=FALSE) -> ()  [unwired: 2 in, 2 out]
              }
            }
          }
        }
        n191 = property on="Progress" class="Clust (strict)"("Visible"=FALSE) -> ()  [unwired: 2 in, 2 out]
      }
      event "Test Name": Mouse Enter {
        # "Populate the ring with the list of tests"
        n192 = event-data() -> ()  [unwired: 1 in, 1 out]
        n193 = call <vilib>:"NT Read String Array.vi"("Name"="TestMode/TestList") -> ("String Array"=w310:string[])  [unwired: 9 in, 1 out]
        n194 = Build Array (concatenate)("Select the test to run...", w310) -> (w309:string[])
        n195 = property on="Test Name" class="Ring (strict)"("Strings []"=w309) -> ()  [unwired: 2 in, 2 out]
      }
      event "Test Name": Value Change {
        w312 = FALSE ("Visible")
        # "Tell the robot the test name to run"
        n196 = event-data() -> ("NewVal"=w316:u16)  [unwired: 1 in]
        n197 = property on="Test Name" class="Ring (strict)"() -> ("Strings []"=w317:string[])  [unwired: 2 in, 2 out]
        n198 = local write "Progress"(T8 {"Test Progress"=0, "Test Progress Text"=""} ("Progress")) -> ()
        n199 = Index Array(array=w317, index=w316) -> (element=w315:string)
        n200 = call <vilib>:"NT Write String.vi"("String"=w315, "Name"="TestMode/TestName") -> ()  [unwired: 9 in, 1 out]
        n201 = property on="Progress" class="Clust (strict)"("Visible"=TRUE) -> ()  [unwired: 2 in, 2 out]
        n202 = property on="Motor" class="Clust (strict)"("Visible"=w312) -> ()  [unwired: 2 in, 2 out]
        n203 = property on="Test Slider" class="Slide (strict)"("Visible"=w312) -> ()  [unwired: 2 in, 2 out]
        n204 = property on="On/Off" class="Bool (strict)"("Visible"=w312) -> ()  [unwired: 2 in, 2 out]
        n205 = property on="Rev/Fwd" class="Clust (strict)"("Visible"=w312) -> ()  [unwired: 2 in, 2 out]
        n206 = property on="Test Ring" class="Ring (strict)"("Visible"=w312) -> ()  [unwired: 2 in, 2 out]
      }
      event "Listbox": Double Click {
        # "Shift clears all"
        # "Update symbols on the listbox"
        n207 = event-data() -> ("PlatMods.Shift"=w320:bool, "Row"=w322:i32)  [unwired: 1 in]
        n208 = case shown="True" w320 {
          tunnel: w322 -> [w326 _]
          tunnel: 1 -> [w325 _]
          frame False {
            n209 = property on="Listbox" class="LstBox (strict)"() -> ("Item Symbols"=w324:i32[])  [unwired: 2 in, 2 out]
            n210 = Replace Array Subset(array=w324, new element=w325, index=w326) -> (w323:i32[])
            n211 = property on="Listbox" class="LstBox (strict)"("Item Symbols"=w323) -> ()  [unwired: 2 in, 2 out]
          }
          frame True {
            w327 = 0 ("Top Row")
            n212 = property on="Listbox" class="LstBox (strict)"() -> ("Number of Rows"=w329:u32)  [unwired: 2 in, 2 out]
            n213 = Initialize Array(0, w329) -> (w328:i32[])
            n214 = property on="Listbox" class="LstBox (strict)"("Top Row"=w327, "Value"=w327, "Item Symbols"=w328) -> ()  [unwired: 2 in, 2 out]
          }
        }
      }
      event "Listbox": Key Down {
        # "Update symbols on the listbox\nLeft and right keys check and uncheck"
        n215 = event-data() -> ("VKey"=w333:T22)  [unwired: 1 in]
        n216 = case shown="\"Left\", \"Right\"" w333 {
          selector: w333 -> [w338 _]
          tunnel: eventvkey."Left" ("VKey") -> [w336 _]
          frame "Left", "Right" {
            n217 = Equal?(x=w336, y=w338) -> (x = y?=w337:bool)
            n218 = Select(t=0, s=w337, f=1) -> (s? t:f=w339:i32)
            n219 = property on="Listbox" class="LstBox (strict)"() -> ("Item Symbols"=w342:i32[])  [unwired: 2 in, 2 out]
            n220 = Replace Array Subset(array=w342, new element=w339, index="Listbox") -> (w341:i32[])
            n221 = property on="Listbox" class="LstBox (strict)"("Item Symbols"=w341) -> ()  [unwired: 2 in, 2 out]
          }
          frame Default {
          }
        }
      }
      event "DB Camera Config": Value Change {
        # "Show or hide the cluster of controls, store in ini file"
        n222 = event-data() -> ("NewVal"=w346:bool)  [unwired: 1 in]
        n223 = case shown="False" w346 {
          tunnel: w345 -> [w355 _]
          tunnel: [w348 w366] -> w344
          tunnel: w343 -> [w347 w366]
          frame False {
            w362 = "Camera"
            w365 = FALSE ("Visible")
            n224 = local read "Camera Settings"() -> (w354:T2)
            n225 = Index Array(array=w355) -> (element=w358:cluster{string[]})  [unwired: 1 in]
            n226 = Unbundle(w354) -> ("Frame Rate"=w353:i32, "Compression"=w352:i32, "Size"=w356:u16)
            n227 = Unbundle(w358) -> (w357:string[])
            n228 = Index Array(array=w357, index=w356) -> (element=w351:string)
            n229 = call-poly <vilib>:"Write Key.vi"("section"=w362, "value"=w351, "key"="Size", "refnum"=w347) -> ("refnum out"=w364:T20)  [unwired: 2 in, 5 out]
            n230 = call-poly <vilib>:"Write Key.vi"("section"=w362, "value"=w353, "key"="FrameRate", "refnum"=w364) -> ("refnum out"=w363:T20)  [unwired: 1 in, 6 out]
            n231 = property on="Camera Settings" class="Clust (strict)"("Visible"=w365) -> ()  [unwired: 2 in, 2 out]
            n232 = local write "DB Camera Config"(w365) -> ()
            n233 = call-poly <vilib>:"Write Key.vi"("section"=w362, "value"=w352, "key"="Compression", "refnum"=w363) -> ("refnum out"=w349:T20)  [unwired: 1 in, 6 out]
            n234 = call <vilib>:"Close Config Data.vi"("refnum"=w349) -> ("file path"=w350:path)  [unwired: 2 in, 8 out]
            n235 = call <vilib>:"Open Config Data.vi"("configuration file path"=w350) -> ("refnum"=w348:T20)  [unwired: 8 in, 2 out]
          }
          frame True {
            n236 = property on="Camera Settings" class="Clust (strict)"("Visible"=TRUE) -> ()  [unwired: 2 in, 2 out]
          }
        }
      }
      event "Camera Settings": Value Change {
        # "Update summary string when any elements of DB camera change"
        n237 = event-data() -> ("NewVal"=w379:T2)  [unwired: 1 in]
        n238 = Index Array(array=w375) -> (element=w374:cluster{string[]})  [unwired: 1 in]
        n239 = Unbundle(w379) -> ("Frame Rate"=w370:i32, "Compression"=w369:i32, "Size"=w372:u16)
        n240 = Unbundle(w374) -> (w373:string[])
        n241 = Index Array(array=w373, index=w372) -> (element=w371:string)
        n242 = Format Into String(format string="%s   %dfps   %d%%", w371, w370, w369) -> (resulting string=w376:string)  [unwired: 2 in, 1 out]
        n243 = Build Array(w376) -> (w377:string[])
        n244 = property on="DB Camera Config" class="Bool (strict)"("Strings [4]"=w377) -> ()  [unwired: 2 in, 2 out]
      }
      event "Motor.Enable": Value Change {
        # "When the test mode otor enable helper is set, update that\ntree row item's value"
        n245 = event-data() -> ("NewVal"=w385:bool)  [unwired: 1 in]
        n246 = Unbundle("Motor") -> ("Value"=w384:dbl)  [unwired: 1 out]
        n247 = Select(t=w384, s=w385, f=0.0) -> (s? t:f=w382:dbl)
        n248 = call <vilib>:"NT Write Number.vi"("Numeric"=w382, "Name"=w381) -> ()  [unwired: 9 in, 1 out]
      }
      event "Test Slider": Value Change {
        # "When the test mode slider helper is set, update that\ntree row item's value"
        n249 = event-data() -> ("NewVal"=w388:dbl)  [unwired: 1 in]
        n250 = call <vilib>:"NT Write Number.vi"("Numeric"=w388, "Name"=w389) -> ()  [unwired: 9 in, 1 out]
      }
      event "On/Off": Value Change {
        # "When the test mode on/off helper value is set, update that\ntree row item's value"
        n251 = event-data() -> ("NewVal"=w393:bool)  [unwired: 1 in]
        n252 = Boolean To (0,1)(Boolean=w393) -> (0, 1=w392:i16)
        n253 = call <vilib>:"NT Write Number.vi"("Numeric"=w392, "Name"=w391) -> ()  [unwired: 9 in, 1 out]
      }
      event "Rev/Fwd": Value Change {
        # "When the test mode helper value for relays is set, update that\ntree row item's value"
        n254 = event-data() -> ("NewVal.Forward"=w401:bool, "NewVal.Reverse"=w400:bool)  [unwired: 1 in]
        n255 = Boolean To (0,1)(Boolean=w401) -> (0, 1=w397:i16)
        n256 = Boolean To (0,1)(Boolean=w400) -> (0, 1=w399:i16)
        n257 = Negate(x=w399) -> (-x=w398:i16)
        n258 = Add(x=w397, y=w398) -> (x+y=w396:i16)
        n259 = call <vilib>:"NT Write Number.vi"("Numeric"=w396, "Name"=w395) -> ()  [unwired: 9 in, 1 out]
      }
      event "Test Ring": Value Change {
        # "When a test mode helper value is selected from the ring,\nset the tree item's variable to the string value"
        n260 = event-data() -> ("NewVal"=w405:u16)  [unwired: 1 in]
        n261 = property on="Test Ring" class="Ring (strict)"() -> ("Strings []"=w406:string[])  [unwired: 2 in, 2 out]
        n262 = Index Array(array=w406, index=w405) -> (element=w404:string)
        n263 = call <vilib>:"NT Write String.vi"("String"=w404, "Name"=w403) -> ()  [unwired: 9 in, 1 out]
      }
      event "Rec Mode": Value Change {
        # "Update globals for recording mode and path to read log from.\nClear when logging and let NetworkTables set path for vision to\nuse."
        n264 = event-data() -> ("NewVal"=w416:enum32{"Stop", "Record", "Playback"})  [unwired: 1 in]
        n265 = global write "WPI_DashboardLogging Global.vi" "Logging Filename"(path "") -> ()
        n266 = case shown="\"Playback\"" w416 {
          tunnel: w415 -> [_ w418 w426]
          tunnel: [_ _ w425] -> w412
          tunnel: [_ _ w424] -> _
          tunnel: w410 -> [_ _ w422]
          tunnel: cluster{i32, i32} {-250, 170} -> [_ _ w421]
          tunnel: [_ _ T23 {"Image Size"=TRUE, "Image Type"=TRUE, "Pixel Value"=TRUE, "ROI Information"=TRUE, "Zoom Factor"=FALSE} ("Image Information Shown:All Elements")] -> w408
          tunnel: [_ _ TRUE ("Zoom Factor")] -> w407
          frame Default {
          }
          frame "Stop", "Record" {
            # "Place Window too"
            n267 = invoke class="VI" method="FP.Close"(reference=w418) -> (reference out=w417:refnum<vi>)  [unwired: 2 in, 2 out]
            n268 = invoke class="VI" method="Abort VI"(reference=w417) -> ()  [unwired: 2 in, 3 out]
          }
          frame "Playback" {
            n269 = call "Open Playback Panel.vi"("Offset"=w421, "DB VI Ref"=w422, "Playback in"=w426) -> ("Playback out"=w423:refnum<vi>)  [unwired: 8 in]
            n270 = register-events(w423) -> (reference out=w425:refnum<event-registration>, error out=w424:errorcluster)  [unwired: 2 in]
          }
        }
        n271 = global write "WPI_DashboardLogging Global.vi" "Recording"(w416) -> ()
        n272 = property on="Camera Image" class="ImageControl"("Image Information Shown"=w408, "Image Information Visible"=w407) -> ()  [unwired: 2 in, 2 out]
        n273 = call <vilib>:"WPI_DashboardNT Log FieldName Cache.vi"("Operation"=enum16{"Lookup/Add", "Index", "Clear"}."Clear") -> ()  [unwired: 8 in, 3 out]
      }
      event Panel Close {
        w427 = enum32{"Stop", "Record", "Playback"}."Stop" ("Rec Mode")
        # "Playback window has been closed, abort"
        n274 = event-data() -> ()  [unwired: 1 in, 4 out]
        n275 = local write "Rec Mode"(w427) -> ()
        n276 = global write "WPI_DashboardLogging Global.vi" "Recording"(w427) -> ()
      }
      event Panel Close {
        # "Abort playback window and ourself"
        n277 = event-data() -> ()  [unwired: 1 in, 4 out]
        n278 = invoke class="VI" method="FP.Close"(reference=w432) -> (reference out=w431:refnum<vi>)  [unwired: 2 in, 2 out]
        n279 = invoke class="VI" method="Abort VI"(reference=w431) -> (error out=w430:errorcluster)  [unwired: 2 in, 2 out]
        n280 = invoke class="VI" method="Abort VI"(error in=w430) -> ()  [unwired: 2 in, 3 out]
      }
      event "Vision": Value Change {
        # "Enable/Disable Compression slider.\nHW USB is hard-coded into the camera"
        n281 = event-data() -> ("NewVal"=w438:u16)  [unwired: 1 in]
        n282 = Equal?(x=w438, y=u32 2 ("milliseconds to wait")) -> (x = y?=w436:bool)
        n283 = Select(t=T24."Disabled and Grayed Out" ("Disabled"), s=w436, f=T24."Enabled" ("Disabled")) -> (s? t:f=w433:T24)
        n284 = property on="Compression" class="Slide (strict)"("DisabledEnum"=w433) -> ()  [unwired: 2 in, 2 out]
      }
    }
  }
  n285 = while {
    tunnel: w38 -> [w441]
    i -> [w444]
    stop <- FALSE stop-if-true
    n286 = Wait (ms)(milliseconds to wait=u32 100) -> ()  [unwired: 1 out]
    n287 = case shown="\"Playback\"" "Rec Mode" {
      tunnel: w444 -> [_ _ w459]
      tunnel: [u32 2829099 ("Base Color") u32 11141120 ("Target Color") w448] -> w440
      frame "Stop", Default {
        # "Reset the color, extra updates don't cost much"
      }
      frame "Record" {
      }
      frame "Playback" {
        # "Playback"
        n288 = Quotient & Remainder(x=w459, y=u32 50 ("milliseconds to wait")) -> (x-y*floor(x/y)=w455:u32)  [unwired: 1 out]
        n289 = Divide(x=w455, y=u32 50 ("milliseconds to wait")) -> (x/y=w452:dbl)
        n290 = Multiply(x=6.283185307179586, y=w452) -> (x*y=w457:dbl)
        n291 = Sine(x=w457) -> (sin(x)=w456:dbl)
        n292 = Absolute Value(x=w456) -> (abs(x)=w449:dbl)
        n293 = call "Interpolate RGB Color.vi"("Proportion"=w449, "Target Color"=u32 30976, "Base Color"=u32 2829099) -> ("Result Color"=w448:u32)  [unwired: 8 in]
      }
    }
    n294 = property class="Pane"(reference=w441, "PaneColor"=w440) -> ()  [unwired: 1 in, 2 out]
  }
  n295 = TCP Create Listener(10:u16 1741 ("timeout ms (25000)")) -> (3:w1:refnum<k5>)  [unwired: 4 in, 2 out]
  n296 = while {
    tunnel: w1 -> [w461]
    stop <- FALSE stop-if-true
    n297 = TCP Wait On Listener(11:w461) -> (4:w460:refnum<k5>)  [unwired: 3 in, 4 out]
    n298 = local write "TCP"(w460) -> ()
  }
  n299 = property on="On/Off" class="Bool (strict)"("Visible"=w6) -> ()  [unwired: 2 in, 2 out]
  n300 = property on="Motor" class="Clust (strict)"("Visible"=w6) -> ()  [unwired: 2 in, 2 out]
  n301 = property on="Progress" class="Clust (strict)"("Visible"=w6) -> ()  [unwired: 2 in, 2 out]
  n302 = property on="Test Ring" class="Ring (strict)"("Visible"=w6) -> ()  [unwired: 2 in, 2 out]
  n303 = property on="Rev/Fwd" class="Clust (strict)"("Visible"=w6) -> ()  [unwired: 2 in, 2 out]
  n304 = property on="Camera Settings" class="Clust (strict)"("Visible"=w6) -> ()  [unwired: 2 in, 2 out]
  n305 = local write "DB Camera Config"(w6) -> ()
  n306 = global write "WPI_DashboardLogging Global.vi" "Recording"(w32) -> ()
  n307 = local write "Rec Mode"(w32) -> ()
